vi "ID Finder.vi"(6 "cluster":T3 {"data[0]"."payload" format="%x"; "data[0]"."timestamp" format="%<%.7X\n%x>T"; "data[0]"."type" items=["CAN Data"=0, "CAN Remote"=1, "CAN Bus Error"=2, "CAN 2.0 Data"=8, "CAN FD Data"=16, "CAN FD+BRS Data"=24, "J1939 Data"=192, "Delay"=224, "Log Trigger"=225, "Start Trigger"=226]; "data[0]"."identifier" format="%x"; "data[1]"."payload" format="%x"; "data[1]"."timestamp" format="%<%.7X\n%x>T"; "data[1]"."type" items=["CAN Data"=0, "CAN Remote"=1, "CAN Bus Error"=2, "CAN 2.0 Data"=8, "CAN FD Data"=16, "CAN FD+BRS Data"=24, "J1939 Data"=192, "Delay"=224, "Log Trigger"=225, "Start Trigger"=226]; "data[1]"."identifier" format="%x"; "data[2]"."payload" format="%x"; "data[2]"."timestamp" format="%<%.7X\n%x>T"; "data[2]"."type" items=["CAN Data"=0, "CAN Remote"=1, "CAN Bus Error"=2, "CAN 2.0 Data"=8, "CAN FD Data"=16, "CAN FD+BRS Data"=24, "J1939 Data"=192, "Delay"=224, "Log Trigger"=225, "Start Trigger"=226]; "data[2]"."identifier" format="%x"; "data[3]"."payload" format="%x"; "data[3]"."timestamp" format="%<%.7X\n%x>T"; "data[3]"."type" items=["CAN Data"=0, "CAN Remote"=1, "CAN Bus Error"=2, "CAN 2.0 Data"=8, "CAN FD Data"=16, "CAN FD+BRS Data"=24, "J1939 Data"=192, "Delay"=224, "Log Trigger"=225, "Start Trigger"=226]; "data[3]"."identifier" format="%x"; "data[4]"."payload" format="%x"; "data[4]"."timestamp" format="%<%.7X\n%x>T"; "data[4]"."type" items=["CAN Data"=0, "CAN Remote"=1, "CAN Bus Error"=2, "CAN 2.0 Data"=8, "CAN FD Data"=16, "CAN FD+BRS Data"=24, "J1939 Data"=192, "Delay"=224, "Log Trigger"=225, "Start Trigger"=226]; "data[4]"."identifier" format="%x"; "data[5]"."payload" format="%x"; "data[5]"."timestamp" format="%<%.7X\n%x>T"; "data[5]"."type" items=["CAN Data"=0, "CAN Remote"=1, "CAN Bus Error"=2, "CAN 2.0 Data"=8, "CAN FD Data"=16, "CAN FD+BRS Data"=24, "J1939 Data"=192, "Delay"=224, "Log Trigger"=225, "Start Trigger"=226]; "data[5]"."identifier" format="%x"; "data[6]"."payload" format="%x"; "data[6]"."timestamp" format="%<%.7X\n%x>T"; "data[6]"."type" items=["CAN Data"=0, "CAN Remote"=1, "CAN Bus Error"=2, "CAN 2.0 Data"=8, "CAN FD Data"=16, "CAN FD+BRS Data"=24, "J1939 Data"=192, "Delay"=224, "Log Trigger"=225, "Start Trigger"=226]; "data[6]"."identifier" format="%x"; "data[7]"."payload" format="%x"; "data[7]"."timestamp" format="%<%.7X\n%x>T"; "data[7]"."type" items=["CAN Data"=0, "CAN Remote"=1, "CAN Bus Error"=2, "CAN 2.0 Data"=8, "CAN FD Data"=16, "CAN FD+BRS Data"=24, "J1939 Data"=192, "Delay"=224, "Log Trigger"=225, "Start Trigger"=226]; "data[7]"."identifier" format="%x"; "data[8]"."payload" format="%x"; "data[8]"."timestamp" format="%<%.7X\n%x>T"; "data[8]"."type" items=["CAN Data"=0, "CAN Remote"=1, "CAN Bus Error"=2, "CAN 2.0 Data"=8, "CAN FD Data"=16, "CAN FD+BRS Data"=24, "J1939 Data"=192, "Delay"=224, "Log Trigger"=225, "Start Trigger"=226]; "data[8]"."identifier" format="%x"}) -> (0 "Data Type":T1 items=["CAN Data"=0, "CAN Remote"=1, "CAN Bus Error"=2, "CAN 2.0 Data"=8, "CAN FD Data"=16, "CAN FD+BRS Data"=24, "J1939 Data"=192, "Delay"=224, "Log Trigger"=225, "Start Trigger"=226], 1 "ID STRING":string, 2 "Payload":u8[](array[numeric]), 3 "Timestamp":timestamp, 4 "Identifier":u32)   [LabVIEW 2023]
uses:
  <vilib>/xnet/xnet.llb/XNET Frame CAN.ctl
  <vilib>/xnet/xnet.llb/XNET Frame Type CAN.ctl
  C:/Elatch-Bench-Test/VIs 64 bits/Users/k90011005/Desktop/Practicas/C#/String-Hexa/bin/Debug/String-Hexa.dll
  VIs 64 bits/Users/k90011005/Desktop/Practicas/C#/String-Hexa/bin/Debug/String-Hexa.dll
panel:
  out "Informacion":string
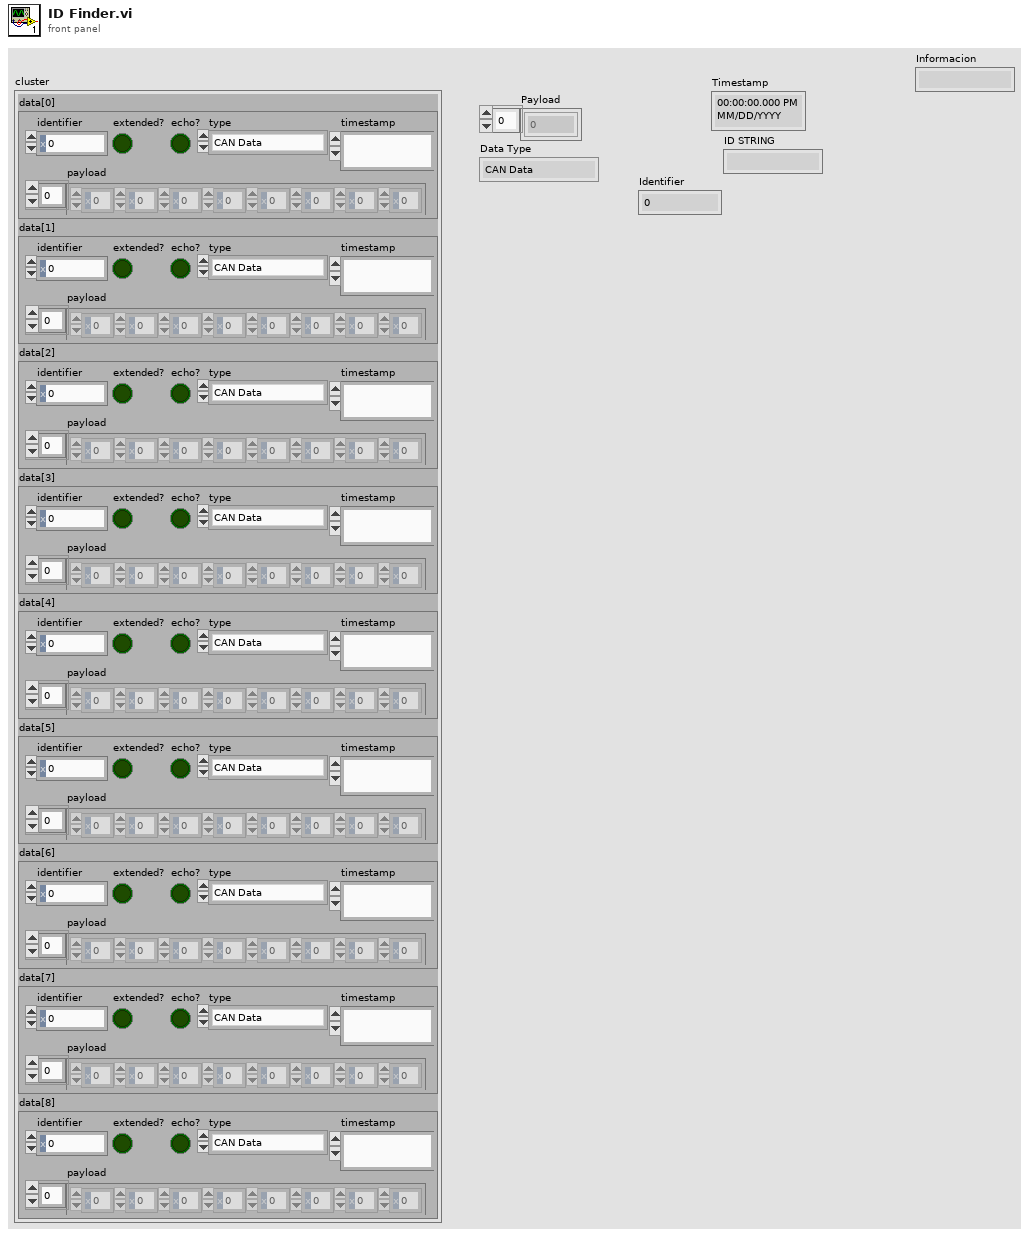
[diagram p1: front panel]
types:
  T1 = typedef "XNET Frame Type CAN.ctl" = u8
  T2 = typedef "XNET Frame CAN.ctl" = cluster{"timestamp":timestamp, "payload":u8[], "identifier":u32, "type":T1, "extended?":bool, "echo?":bool}
  T3 = cluster{"data[0]":T2, "data[1]":T2, "data[2]":T2, "data[3]":T2, "data[4]":T2, "data[5]":T2, "data[6]":T2, "data[7]":T2, "data[8]":T2}
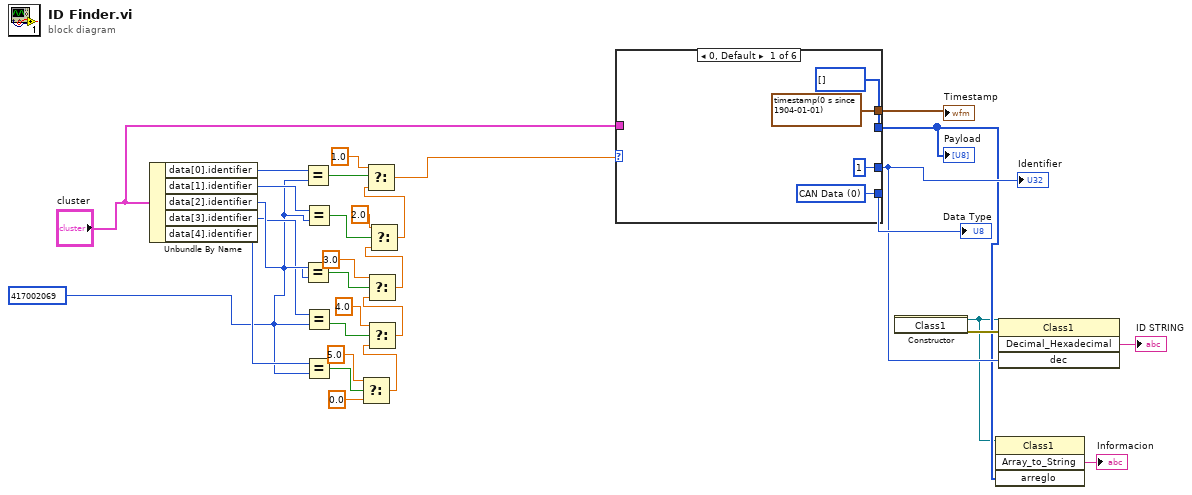
[diagram p0: block diagram]
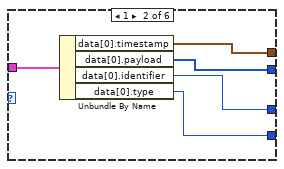
[diagram p2: hidden frame]
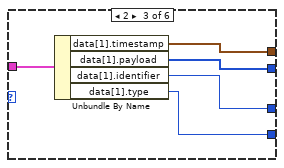
[diagram p3: hidden frame]
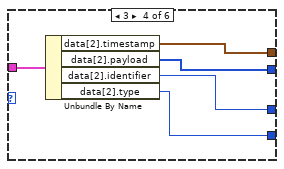
[diagram p4: hidden frame]
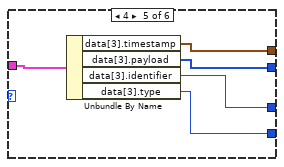
[diagram p5: hidden frame]
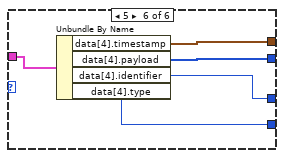
[diagram p6: hidden frame]
diagram:
  w22 = u32 417002069 ("y")
  n1 = Unbundle By Name("cluster") -> ("data[0].identifier"=w31:u32, "data[1].identifier"=w26:u32, "data[2].identifier"=w25:u32, "data[3].identifier"=w24:u32, "data[4].identifier"=w23:u32)
  n2 = Equal?(x=w31, y=w22) -> (x = y?=w30:bool)
  n3 = Equal?(x=w25, y=w22) -> (x = y?=w16:bool)
  n4 = Equal?(x=w26, y=w22) -> (x = y?=w17:bool)
  n5 = Equal?(x=w24, y=w22) -> (x = y?=w15:bool)
  n6 = Equal?(x=w23, y=w22) -> (x = y?=w14:bool)
  n7 = Select(t=5.0, s=w14, f=0.0) -> (s? t:f=w18:dbl)
  n8 = Select(t=4.0, s=w15, f=w18) -> (s? t:f=w19:dbl)
  n9 = Select(t=3.0, s=w16, f=w19) -> (s? t:f=w20:dbl)
  n10 = Select(t=2.0, s=w17, f=w20) -> (s? t:f=w21:dbl)
  n11 = Select(t=1.0, s=w30, f=w21) -> (s? t:f=w28:dbl)
  n12 = case shown="0, Default" w28 {
    tunnel: "cluster" -> [_ w40 w45 w50 w55 w60]
    tunnel: [timestamp(0 s since 1904-01-01) ("timestamp") w39 w44 w49 w54 w59] -> w8
    tunnel: [u8[] [] ("payload") w38 w43 w48 w53 w58] -> w3
    tunnel: [u32 1 ("identifier") w37 w42 w47 w52 w57] -> w5
    tunnel: [w32 w36 w41 w46 w51 w56] -> w7
    frame 0, Default {
      w32 = T1 0 items=["CAN Data"=0, "CAN Remote"=1, "CAN Bus Error"=2, "CAN 2.0 Data"=8, "CAN FD Data"=16, "CAN FD+BRS Data"=24, "J1939 Data"=192, "Delay"=224, "Log Trigger"=225, "Start Trigger"=226] ("type")
    }
    frame 1 {
      n13 = Unbundle By Name(w40) -> ("data[0].timestamp"=w39:timestamp, "data[0].payload"=w38:u8[], "data[0].identifier"=w37:u32, "data[0].type"=w36:T1)
    }
    frame 2 {
      n14 = Unbundle By Name(w45) -> ("data[1].timestamp"=w44:timestamp, "data[1].payload"=w43:u8[], "data[1].identifier"=w42:u32, "data[1].type"=w41:T1)
    }
    frame 3 {
      n15 = Unbundle By Name(w50) -> ("data[2].timestamp"=w49:timestamp, "data[2].payload"=w48:u8[], "data[2].identifier"=w47:u32, "data[2].type"=w46:T1)
    }
    frame 4 {
      n16 = Unbundle By Name(w55) -> ("data[3].timestamp"=w54:timestamp, "data[3].payload"=w53:u8[], "data[3].identifier"=w52:u32, "data[3].type"=w51:T1)
    }
    frame 5 {
      n17 = Unbundle By Name(w60) -> ("data[4].timestamp"=w59:timestamp, "data[4].payload"=w58:u8[], "data[4].identifier"=w57:u32, "data[4].type"=w56:T1)
    }
  }
  "Timestamp" <- w8
  "Payload" <- w3
  "Identifier" <- w5
  "Data Type" <- w7
  n18 = constructor class="Class1"() -> (reference out=w1:refnum<k24>, error out=w6:errorcluster)  [unwired: 3 in, 1 out]
  n19 = invoke class="Class1" method="Array_to_String"(reference=w1, "arreglo"=w3) -> ("Array_to_String"=→"Informacion":string)  [unwired: 2 in, 3 out]
  n20 = invoke class="Class1" method="Decimal_Hexadecimal"(reference=w1, error in=w6, "dec"=w5) -> ("Decimal_Hexadecimal"=→"ID STRING":string)  [unwired: 1 in, 3 out]
